vi "disdrometer_serialcomm.vi"(6 "UserCommand":string="RS00001", 8 "Error In":errorcluster, 10 "CommandToSend":T1=enum."UserCommand", 11 "Resource Name":refnum<visa-resource-name>) -> (0 "Error Out":errorcluster, 1 "Success":bool, 2 "Poll Response":string)   [LabVIEW 2018]
doc: "Polls the Thies Clima disdrometer to request data. The running total of accumulation can be reset to zero with the boolean \"Reset Accum\" input."
uses:
  Disdrometer_Message_To_Send_Enum.ctl
  <vilib>/Instr/_visa.llb/VISA Configure Serial Port (Instr).vi
panel:
  in  "Device ID":string="00"
  out "Bytes Read":u32
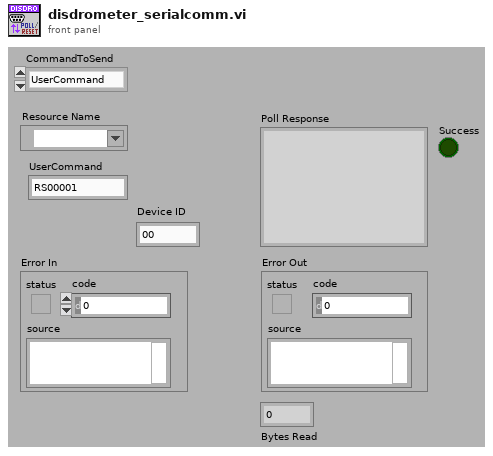
[diagram p1: front panel]
types:
  T1 = typedef "Disdrometer_Message_To_Send_Enum.ctl" = enum16{"None", "ResetAccum", "ResetDisdrom", "UserCommand"}
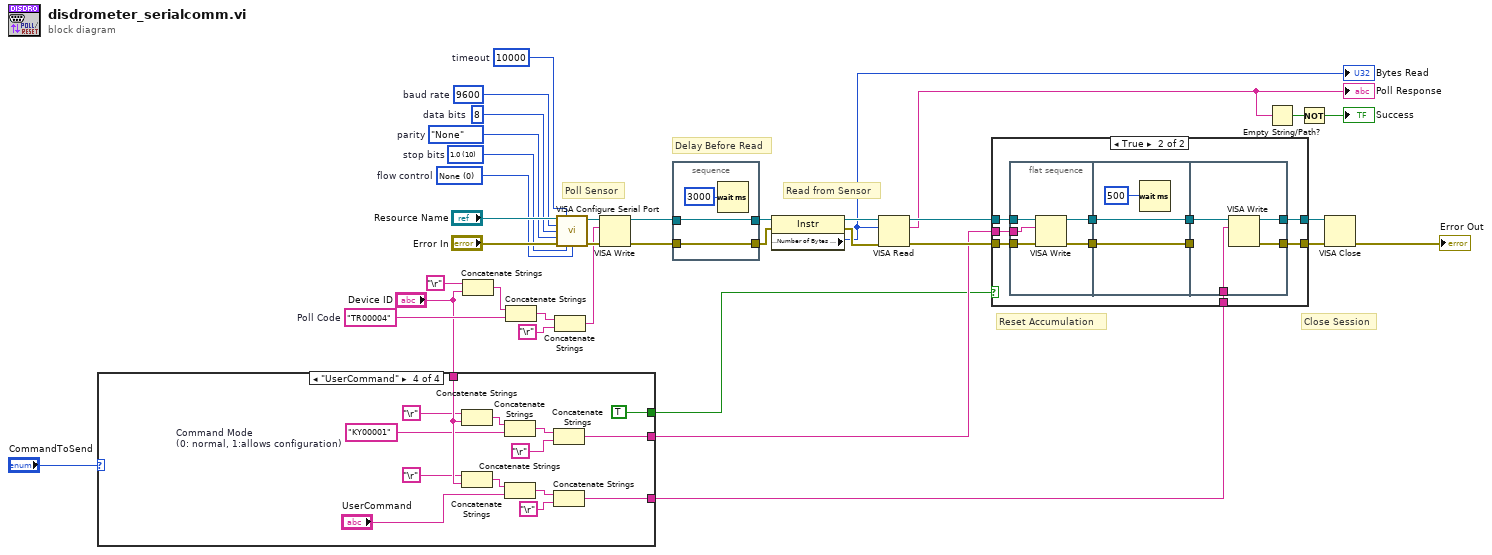
[diagram p0: block diagram]
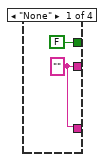
[diagram p2: hidden frame]
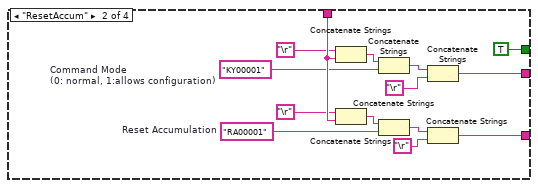
[diagram p3: hidden frame]
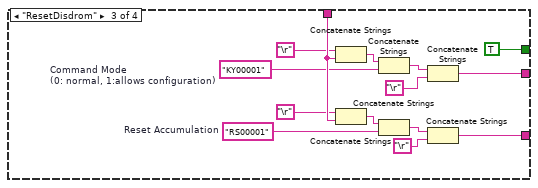
[diagram p4: hidden frame]
diagram:
  w19 = u32 10000  # timeout
  w11 = "TR00004"  # Poll Code
  w17 = u16 0 items=["None", "XON/XOFF", "RTS/CTS", "XON/XOFF & RTS/CTS", "DTR/DSR", "XON/XOFF & DTR/DSR"]  # flow control
  w18 = u16 10 items=["1.0"=10, "1.5"=15, "2.0"=20]  # stop bits
  w20 = enum16{"None", "Odd", "Even", "Mark", "Space"}."None"  # parity
  w21 = u16 8  # data bits
  w22 = u32 9600  # baud rate
  # "Reset Accumulation"
  # "Close Session"
  # "Delay Before Read"
  # "Read from Sensor"
  # "Poll Sensor"
  n1 = case shown="\"UserCommand\"" "CommandToSend" {
    tunnel: "Device ID" -> [_ w47 w61 w75]
    tunnel: [w37 w45 w59 w73] -> w9
    tunnel: [w37 w44 w58 w72] -> w8
    tunnel: [FALSE ("Send Command") TRUE ("Send Command") TRUE ("Send Command") TRUE ("Send Command")] -> w1
    frame "None" {
      w37 = ""
    }
    frame "ResetAccum" {
      w50 = "RA00001"  # Reset Accumulation
      w46 = "KY00001"  # Command Mode (0: normal, 1:allows configuration)
      n2 = Concatenate Strings("\r", w47) -> (w49:string)
      n3 = Concatenate Strings("\r", w47) -> (w52:string)
      n4 = Concatenate Strings(w49, w46) -> (w48:string)
      n5 = Concatenate Strings(w52, w50) -> (w51:string)
      n6 = Concatenate Strings(w48, "\r") -> (w45:string)
      n7 = Concatenate Strings(w51, "\r") -> (w44:string)
    }
    frame "ResetDisdrom" {
      w64 = "RS00001"  # Reset Accumulation
      w60 = "KY00001"  # Command Mode (0: normal, 1:allows configuration)
      n8 = Concatenate Strings("\r", w61) -> (w63:string)
      n9 = Concatenate Strings("\r", w61) -> (w66:string)
      n10 = Concatenate Strings(w63, w60) -> (w62:string)
      n11 = Concatenate Strings(w66, w64) -> (w65:string)
      n12 = Concatenate Strings(w62, "\r") -> (w59:string)
      n13 = Concatenate Strings(w65, "\r") -> (w58:string)
    }
    frame "UserCommand" {
      w74 = "KY00001"  # Command Mode (0: normal, 1:allows configuration)
      n14 = Concatenate Strings("\r", w75) -> (w77:string)
      n15 = Concatenate Strings("\r", w75) -> (w80:string)
      n16 = Concatenate Strings(w77, w74) -> (w76:string)
      n17 = Concatenate Strings(w80, "UserCommand") -> (w79:string)
      n18 = Concatenate Strings(w76, "\r") -> (w73:string)
      n19 = Concatenate Strings(w79, "\r") -> (w72:string)
    }
  }
  n20 = Concatenate Strings("\r", "Device ID") -> (w14:string)
  n21 = Concatenate Strings(w14, w11) -> (w13:string)
  n22 = Concatenate Strings(w13, "\r") -> (w12:string)
  n23 = call-poly "VISA Configure Serial Port"("VISA resource name"="Resource Name", "timeout (10sec)"=w19, "baud rate (9600)"=w22, "data bits (8)"=w21, "parity (0:none)"=w20, "error in (no error)"="Error In", "stop bits (10: 1 bit)"=w18, "flow control (0:none)"=w17) -> ("VISA resource name out"=w32:refnum<visa-resource-name>, "error out"=w31:errorcluster)  [unwired: 1 in, 5 out]
  n24 = VISA Write(VISA resource name=w32, write buffer=w12, error in (no error)=w31) -> (VISA resource name out=w27:refnum<visa-resource-name>, error out=w25:errorcluster)  [unwired: 1 out]
  n25 = stacked-sequence {
    tunnel: w25 -> [w83]
    tunnel: [w83] -> w26
    tunnel: w27 -> [w82]
    tunnel: [w82] -> w28
    frame #0 {
      n26 = Wait (ms)(milliseconds to wait=u32 3000 ("delay before read (ms)")) -> ()  [unwired: 1 out]
    }
  }
  n27 = property class="Instr"(reference=w28, error in=w26) -> (reference out=w29:refnum<visa-resource-name>, error out=w30:errorcluster, "Serial Settings:Number of Bytes at Serial Port"=w5:u32)
  "Bytes Read" <- w5
  n28 = VISA Read(VISA resource name=w29, byte count=w5, error in (no error)=w30) -> (VISA resource name out=w33:refnum<visa-resource-name>, read buffer=w15:string, error out=w34:errorcluster)  [unwired: 1 out]
  "Poll Response" <- w15
  n29 = case shown="True" w1 {
    tunnel: [w85 w87] -> w35
    tunnel: w33 -> [w85 w94]
    tunnel: [w84 w86] -> w36
    tunnel: w34 -> [w84 w93]
    tunnel: w9 -> [_ w95]
    tunnel: w8 -> [_ w88]
    frame False {
    }
    frame True {
      n30 = flat-sequence {
        tunnel: w95 -> [w100]
        tunnel: w94 -> [w99]
        tunnel: w93 -> [w98]
        tunnel: [w97] -> w91
        tunnel: [w96] -> w89
        tunnel: [w103] -> w92
        tunnel: w91 -> [w103]
        tunnel: [w102] -> w90
        tunnel: w89 -> [w102]
        tunnel: w92 -> [w107]
        tunnel: w90 -> [_]
        tunnel: w88 -> [w106]
        tunnel: [w105] -> w87
        tunnel: [w104] -> w86
        frame #0 {
          n31 = VISA Write(VISA resource name=w99, write buffer=w100, error in (no error)=w98) -> (VISA resource name out=w97:refnum<visa-resource-name>, error out=w96:errorcluster)  [unwired: 1 out]
        }
        frame #1 {
          n32 = Wait (ms)(milliseconds to wait=u32 500 ("delay before read (ms)")) -> ()  [unwired: 1 out]
        }
        frame #2 {
          n33 = VISA Write(VISA resource name=w107, write buffer=w106) -> (VISA resource name out=w105:refnum<visa-resource-name>, error out=w104:errorcluster)  [unwired: 1 in, 1 out]
        }
      }
    }
  }
  n34 = Empty String/Path?(string/path=w15) -> (empty?=w16:bool)
  n35 = Not(x=w16) -> (.not. x?=→"Success":bool)
  n36 = VISA Close(VISA resource name=w35, error in (no error)=w36) -> (error out=→"Error Out":errorcluster)
